vi "createpath.vi"(8 "header":string, 11 "base path":path) -> (3 "appended path":path)   [LabVIEW 2012]
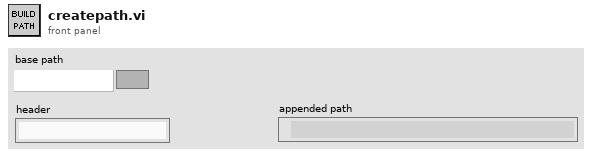
[diagram p1: front panel]
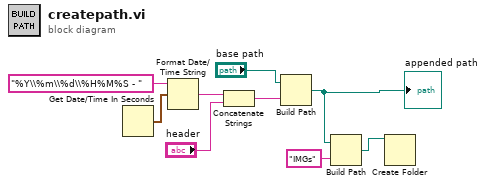
[diagram p0: block diagram]
diagram:
  n1 = Get Date/Time In Seconds() -> (seconds since 1Jan1904=w9:timestamp)
  n2 = Format Date/Time String(time format string (%c)="%Y\\%m\\%d\\%H%M%S - ", seconds (now)=w9) -> (date/time string=w8:string)  [unwired: 1 in]
  n3 = Concatenate Strings(w8, "header") -> (w4:string)
  n4 = Build Path(base path="base path", name or relative path=w4) -> (appended path=w1:path)
  "appended path" <- w1
  n5 = Build Path(base path=w1, name or relative path="IMGs") -> (appended path=w2:path)
  n6 = Create Folder(path (use dialog)=w2) -> ()  [unwired: 2 in, 3 out]
